vi "thermodiodeMain.vi"() -> ()   [LabVIEW 2023]
uses:
  <vilib>/Utility/file.llb/Write Delimited Spreadsheet (DBL).vi
  <vilib>/Analysis/NI_AALBase.lvlib
panel:
  out "temperature 2":dbl format="%0.2f"
  out "standard deviation":dbl format="%0.2f"
  out "mean":dbl format="%0.6e"
  in  "file path (dialog if empty)":path
  in  "stop":bool
  out "Temperature (deg C)":dbl(graph)
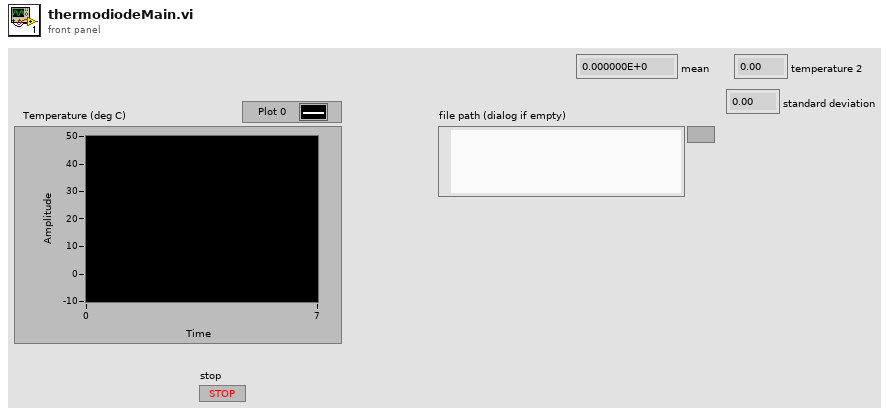
[diagram p1: front panel]
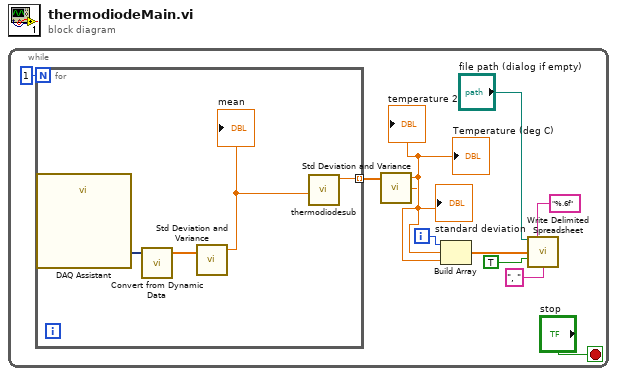
[diagram p0: block diagram]
diagram:
  n1 = while {
    i -> [w10]
    stop <- "stop" stop-if-true
    n2 = for {
      N: 1 -> [_]
      tunnel: [w13] -> w5 mode=indexing
      n3 = call "DAQ Assistant"() -> ("data"=w15:dynamicdata)  [unwired: 17 in, 2 out]
      n4 = call "Convert from Dynamic Data"("Dynamic Data Type"=w15) -> ("Array"=w14:dbl[])  [unwired: 3 in]
      n5 = call <vilib>:"Std Deviation and Variance.vi"("X"=w14) -> ("mean"=w12:dbl)  [unwired: 1 in, 2 out]
      "mean" <- w12
      n6 = call "thermodiodesub.vi"("voltage"=w12) -> ("temperature C"=w13:dbl)  [unwired: 10 in]
    }
    n7 = call <vilib>:"Std Deviation and Variance.vi"("X"=w5) -> ("mean"=w4:dbl, "standard deviation"=w3:dbl)  [unwired: 1 in, 1 out]
    "Temperature (deg C)" <- w4
    "standard deviation" <- w3
    "temperature 2" <- w4
    n8 = Build Array(w10, w4, w3) -> (w9:dbl[])
    n9 = call-poly <vilib>:"Write Delimited Spreadsheet.vi"("file path (dialog if empty)"="file path (dialog if empty)", "format (%.3f)"="%.6f", "1D data"=w9, "append to file? (new file:F)"=TRUE, "delimiter (\\t)"=", " ("delimiter (\\t)")) -> ()  [unwired: 9 in, 2 out]
  }
